vi "Read Tag.vi"(5 "Override type":cluster{"ID":string, "Type":T1}, 6 "IFD Info":T3(c390), 8 "error in (no error)":errorcluster, 10 "Tag ID":T2=254, 11 "TIFF Reader in":refnum<class "TIFF Reader.lvclass">) -> (0 "error out":errorcluster, 1 "Tag found?":bool, 2 "Tag Data":variant, 3 "TIFF Reader out":refnum<class "TIFF Reader.lvclass">)   [LabVIEW 2020, in "LV Tiff.lvlib" / "TIFF Reader.lvclass"]
uses:
  TIFF Reader.lvclass
  _Helpers/Tiff Data Type.ctl
  _Helpers/Tiff Tags.ctl
  TIFF Reader.lvclass/TIFF Reader.ctl
  LV Tiff.lvlib
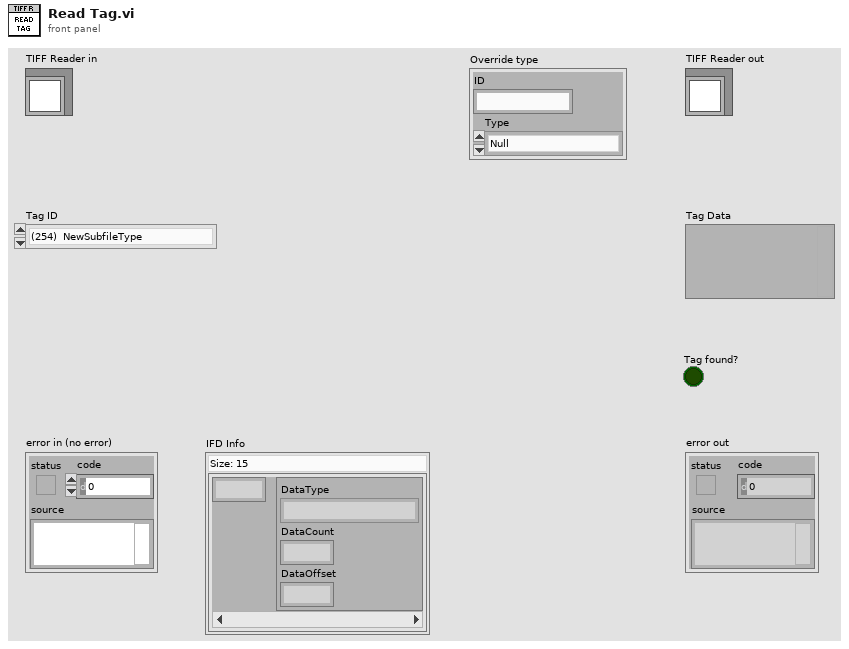
[diagram p1: front panel]
types:
  T1 = typedef "LV Tiff.lvlib/Tiff Data Type.ctl" = enum16{"Null", "BYTE", "ASCII", "SHORT", "LONG", "RATIONAL", "SBYTE", "UNDEFINE", "SSHORT", "SLONG", "SRATIONAL", "FLOAT", "DOUBLE"}
  T2 = typedef "LV Tiff.lvlib/Tiff Tags.ctl" = u16
  T3 = map{u16, cluster{"DataType":T1, "DataCount":u32, "DataOffset":u32}}
  T4 = enum16{"big-endian, network order", "native, host order", "little-endian"}
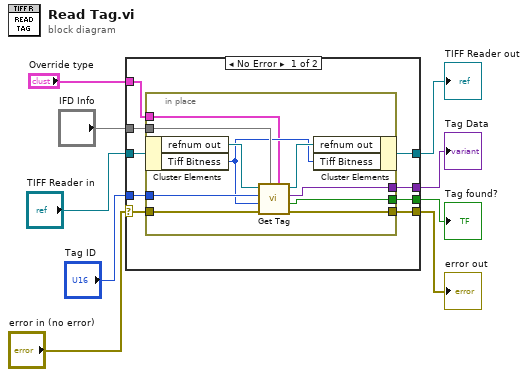
[diagram p0: block diagram]
diagram:
  n1 = case shown="No Error" "error in (no error)" {
    selector: "error in (no error)" -> [w16 w30]
    tunnel: [w15 w30] -> w8
    tunnel: [w17 w29] -> w6
    tunnel: "TIFF Reader in" -> [w18 w29]
    tunnel: "IFD Info" -> [w14 _]
    tunnel: "Tag ID" -> [w13 _]
    tunnel: [w12 _] -> w3
    tunnel: [w11 _] -> w2
    tunnel: "Override type" -> [w10 _]
    frame No Error {
      n2 = in-place {
        in-place-border: w16 -> [w28]
        in-place-border: [w27] -> w15
        in-place-border: w14 -> [w24]
        in-place-border: w13 -> [w23]
        in-place-border: [w22] -> w12
        in-place-border: [w20] -> w11
        in-place-border: w10 -> [w19]
        n3 = in-place-cluster #1(w18) -> ("refnum out"=w26:refnum<file>, "Tiff Bitness"=w21:T4)
        n4 = call "Get Tag.vi"("Override type"=w19, "IFDO"=w24, "error in 2"=w28, "byte order (0:big-endian, network order)"=w21, "Tag ID"=w23, "File Refnum"=w26) -> ("error out"=w27:errorcluster, "Tag found?"=w20:bool, "Data"=w22:variant, "refnum out"=w25:refnum<file>)  [unwired: 2 in]
        n5 = in-place-cluster #1("refnum out"=w25, "Tiff Bitness"=w21) -> (w17:refnum<class "TIFF Reader.lvclass">)
      }
    }
    frame Error {
    }
  }
  "error out" <- w8
  "TIFF Reader out" <- w6
  "Tag Data" <- w3
  "Tag found?" <- w2
